vi "Pump Status.vi"(8 "error in (no error)":errorcluster, 11 "Ismatech 3 Channel Settings In":T1={"VISA resource name"="", "Pump Number"=1, "Channel Number"=0, "Simulated?"=TRUE, "Reverse?"=FALSE} {"Channel Number" min=0 max=3; "Pump Number" min=1 max=9}) -> (0 "error out":errorcluster, 1 "Connection Error":bool, 2 "Pump On?":enum16{"Off", "On", "Not Initialized"}(ring), 3 "Ismatech 3 Channel Settings Out":T1={"VISA resource name"="", "Pump Number"=1, "Channel Number"=0, "Simulated?"=TRUE, "Reverse?"=FALSE} {"Channel Number" min=0 max=3; "Pump Number" min=1 max=9}, 4 "RPM":dbl)   [LabVIEW 2018, in "Ismatec 4308.lvlib"]
uses:
  Ismatec 4308.lvlib
  Ismatec 4083.ctl
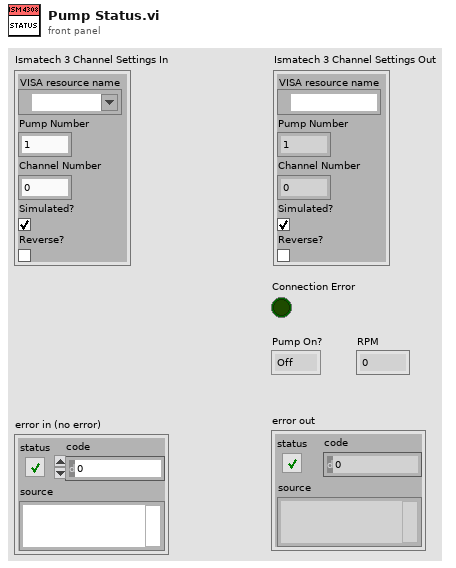
[diagram p1: front panel]
types:
  T1 = typedef "Ismatec 4308.lvlib/Ismatec 4083.ctl" = cluster{"VISA resource name":refnum<visa-resource-name>, "Pump Number":i16, "Channel Number":i16, "Simulated?":bool, "Reverse?":bool}
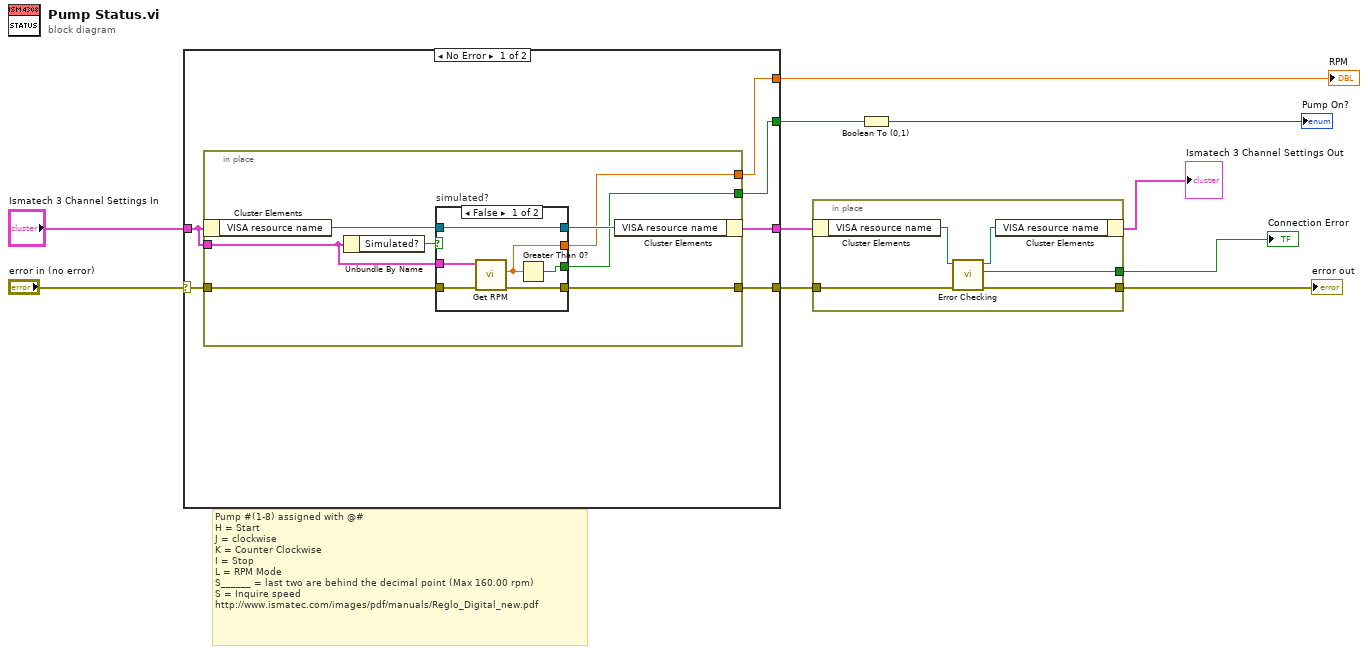
[diagram p0: block diagram]
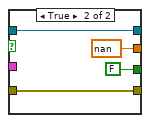
[diagram p2: hidden frame]
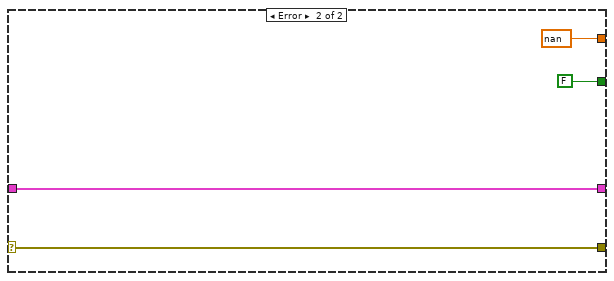
[diagram p3: hidden frame]
diagram:
  # "Pump #(1-8) assigned with @#\nH = Start\nJ = clockwise\nK = Counter Clockwise\nI = Stop\nL = RPM Mode\nS______ = last two are behind the decimal point (Max 160.00 rpm)\nS = Inquire speed\nhttp://www.ismatec.com/images/pdf/manuals/Reglo_Digital_new.pdf"
  n1 = case shown="No Error" "error in (no error)" {
    selector: "error in (no error)" -> [w15 w38]
    tunnel: [w16 w38] -> w9
    tunnel: [w13 w37] -> w6
    tunnel: "Ismatech 3 Channel Settings In" -> [w14 w37]
    tunnel: [w11 FALSE] -> w7
    tunnel: [w12 nan ("RPM")] -> w1
    frame No Error {
      n2 = in-place {
        in-place-border: [w23] -> w16
        in-place-border: w14 -> [w18]
        in-place-border: w15 -> [w22]
        in-place-border: [w19] -> w12
        in-place-border: [w17] -> w11
        n3 = in-place-cluster #1(w14) -> ("VISA resource name"=w20:refnum<visa-resource-name>)
        n4 = Unbundle By Name(w18) -> ("Simulated?"=w24:bool)
        n5 = case "simulated?" shown="False" w24 {
          tunnel: [w29 w33] -> w23
          tunnel: [w30 w34] -> w21
          tunnel: w20 -> [w30 w34]
          tunnel: w22 -> [w26 w33]
          tunnel: [w25 nan ("RPM")] -> w19
          tunnel: w18 -> [w28 _]
          tunnel: [w27 FALSE] -> w17
          frame False {
            n6 = call "Get RPM.vi"("error in (no error)"=w26, "Ismatech 3 Channel Settings In"=w28) -> ("error out"=w29:errorcluster, "RPM"=w25:dbl)  [unwired: 7 in, 1 out]
            n7 = Greater Than 0?(x=w25) -> (x > 0?=w27:bool)
          }
          frame True {
          }
        }
        n8 = in-place-cluster #1("VISA resource name"=w21) -> (w13:T1)
      }
    }
    frame Error {
    }
  }
  "RPM" <- w1
  n9 = in-place {
    in-place-border: w9 -> [w43]
    in-place-border: [w40] -> w5
    in-place-border: [w39] -> w4
    n10 = in-place-cluster #2(w6) -> ("VISA resource name"=w42:refnum<visa-resource-name>)
    n11 = call "Error Checking.vi"("error in (no error)"=w43, "VISA resource name"=w42) -> ("error out"=w39:errorcluster, "Connection Error"=w40:bool, "VISA resource name"=w41:refnum<visa-resource-name>)  [unwired: 7 in]
    n12 = in-place-cluster #2("VISA resource name"=w41) -> (→"Ismatech 3 Channel Settings Out":T1)
  }
  "error out" <- w4
  "Connection Error" <- w5
  n13 = Boolean To (0,1)(Boolean=w7) -> (0, 1=→"Pump On?":i16)
